vi "oa_Process Counter Data (1 Tach).vi"(7 "reset?(True)":bool=TRUE, 8 "error in (no error)":errorcluster, 9 "vibration signal duration [s]":dbl format="%0.2f", 11 "digital tach info":T1={"tacho counts"=[], "counter timebase [Hz]"=20000000.0, "counter task type"=enum."event counting", "counter digit (32)"=32}) -> (0 "error out (no error)":errorcluster, 3 "digital tach info (DBL)":T2={"pulse positions [s]"=[], "counter timebase [Hz]"=20000000.0, "counter task type"=enum."event counting", "counter digit"=32})   [LabVIEW 2017, in "SoundVib_TachProcess.lvlib"]
uses:
  <vilib>/addons/Sound and Vibration/Order Analysis/Tach Process/SoundVib_TachProcess.lvlib
  <vilib>/addons/Sound and Vibration/Order Analysis/Tach Process/SubVIs/digital tach info.ctl
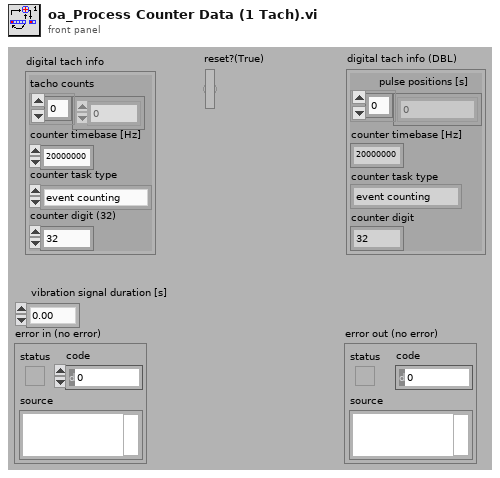
[diagram p1: front panel]
types:
  T1 = typedef "SoundVib_TachProcess.lvlib/digital tach info.ctl" = cluster{"tacho counts":i64[], "counter timebase [Hz]":dbl, "counter task type":enum16{"period measurement", "event counting"}, "counter digit (32)":i32}
  T2 = cluster{"pulse positions [s]":dbl[], "counter timebase [Hz]":dbl, "counter task type":enum16{"period measurement", "event counting"}, "counter digit":i32}
  T3 = cluster{"time offset":dbl, "event count":u64, "time without pulse":ext}
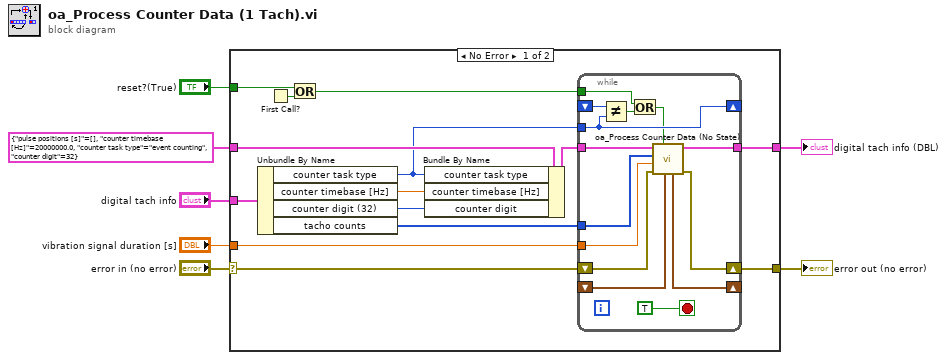
[diagram p0: block diagram]
diagram:
  n1 = case shown="No Error" "error in (no error)" {
    selector: "error in (no error)" -> [w9 w37]
    tunnel: [w8 w37] -> w6
    tunnel: "digital tach info" -> [w21 _]
    tunnel: [w19 w36] -> w4
    tunnel: "vibration signal duration [s]" -> [w20 _]
    tunnel: "reset?(True)" -> [w17 _]
    tunnel: T2 {"pulse positions [s]"=[], "counter timebase [Hz]"=20000000.0, "counter task type"=enum."event counting", "counter digit"=32} ("digital tach info") -> [w11 w36]
    frame No Error {
      n2 = Unbundle By Name(w21) -> ("counter task type"=w10:enum16{"period measurement", "event counting"}, "counter timebase [Hz]"=w12:dbl, "counter digit (32)"=w13:i32, "tacho counts"=w15:i64[])
      n3 = First Call?() -> (First Call?: T/F=w18:bool)
      n4 = Or(x=w17, y=w18) -> (x .or. y?=w16:bool)
      n5 = Bundle By Name(cluster=w11, "counter task type"=w10, "counter timebase [Hz]"=w12, "counter digit"=w13) -> (w14:T2)
      n6 = while {
        tunnel: w10 -> [w31]
        shift-right: [w31] -> _
        shift-left: _ -> [w34]
        tunnel: w16 -> [w32]
        shift-right: [w24] -> _
        shift-left: _ -> [w25]
        tunnel: w14 -> [w30]
        tunnel: w20 -> [w26]
        tunnel: [w29] -> w19
        tunnel: w15 -> [w27]
        shift-right: [w22] -> w8
        shift-left: w9 -> [w23]
        stop <- TRUE stop-if-true
        n7 = Not Equal?(x=w34, y=w31) -> (x != y?=w33:bool)
        n8 = Or(x=w32, y=w33) -> (x .or. y?=w28:bool)
        n9 = call <vilib>:"oa_Process Counter Data (No State).vi"("state in"=w25, "reset"=w28, "error in (no error)"=w23, "vibration signal duration [s]"=w26, "tacho counts"=w27, "digital tach info in"=w30) -> ("error out"=w22:errorcluster, "digital tach info out"=w29:T2, "state out"=w24:T3)  [unwired: 3 in]
      }
    }
    frame Error {
    }
  }
  "error out (no error)" <- w6
  "digital tach info (DBL)" <- w4
